vi "logic_block.vi"(1 "C":T1, 2 "B":bool, 3 "A":bool) -> (0 "R":bool)   [LabVIEW 2013]
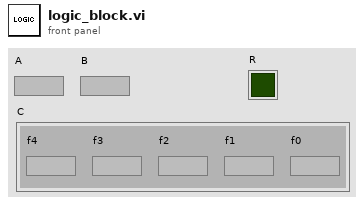
[diagram p1: front panel]
types:
  T1 = cluster{"f4":bool, "f3":bool, "f2":bool, "f1":bool, "f0":bool}
  T2 = cluster{bool, bool, bool, bool, bool, bool, bool, bool, bool, bool}
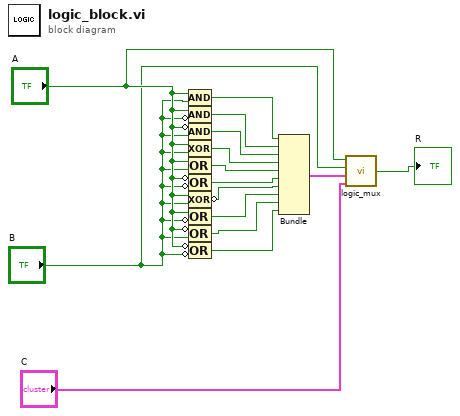
[diagram p0: block diagram]
diagram:
  n1 = Compound Arithmetic op=AND("A", "B") -> (w15:bool)
  n2 = Compound Arithmetic op=AND("A", invert "B") -> (w14:bool)
  n3 = Compound Arithmetic op=AND(invert "A", "B") -> (w12:bool)
  n4 = Compound Arithmetic op=XOR("A", "B") -> (w13:bool)
  n5 = Compound Arithmetic op=OR("A", "B") -> (w11:bool)
  n6 = Compound Arithmetic op=OR(invert "A", invert "B") -> (w10:bool)
  n7 = Compound Arithmetic op=XOR("A", "B") -> (invert w8:bool)
  n8 = Compound Arithmetic op=OR("A", invert "B") -> (w9:bool)
  n9 = Compound Arithmetic op=OR(invert "A", "B") -> (w7:bool)
  n10 = Compound Arithmetic op=OR(invert "A", invert "B") -> (w6:bool)
  n11 = Bundle(w15, w14, w12, w13, w11, w10, w8, w9, w7, w6) -> (w3:T2)  [unwired: 1 in]
  n12 = call "logic_mux.vi"("C"="C", "R-1"=w3, "B"="B", "A"="A") -> ("R"=→"R":bool)
